vi "RT Loop - Analyze Acceleration_V2_CSV.vi"(7 "testing":bool, 8 "error in (no error)":errorcluster, 9 "Acceleration RT FIFO In":T2, 10 "FPGA VI Reference Out 2":refnum<k20>, 11 "Message Queue":refnum<queue>) -> (1 "Acceleration RT FIFO Out":T2)   [LabVIEW 2017]
doc: "Read and analyze acceleration waveform data from FPGA via DMA FIFO. If the acceleration is over the limit, then send the acceleration waveform data to the Log Data Loop."
uses:
  UI Error Handlers/support/Message Queue/Message Cluster.ctl
  controls/Acceleration RT FIFO Reference.ctl
  Control 1.ctl
  data_sav.ctl
  Globals/Global - All RT Loop Stop.vi
  <vilib>/Utility/file.llb/Write Delimited Spreadsheet (DBL).vi
  Globals/Global - Configuration Options.vi
  <vilib>/Utility/error.llb/Error Cluster From Error Code.vi
  <vilib>/rvi/errors/niLvFpgaAdjustHostInterfaceError.vi
  <vilib>/Utility/file.llb/Write Delimited Spreadsheet (string).vi
  <vilib>/rvi/interface/nirviMethod/nirviMethod.xnode
  <vilib>/FPGAPlugInAG/Dynamic/niLvFpga_ReadFifo_Dynamic.vi
  <vilib>/rvi/errors/niLvFpgaMergeErrorWithErrorCode.vi
  UI Error Handlers/support/Message Queue/Message Queue.lvlib
panel:
  out "size(s)":i32
  out "Cluster":cluster{"Array":T1[], "AVI Path":path}={"Array"=[], "AVI Path"=path "u:/data_log"}
  out "Free Physical Memory or Largest Contiguous Memory (bytes)":i64(graph)
  out "error out":errorcluster
  out "x-y":u32
  out "G1 status":cluster{"G1 trigger":bool}
  out "G1 status.G1 trigger":bool
  out "sta":bool
  out "logical OR":bool
  in  "Data Rate (Hz)":dbl
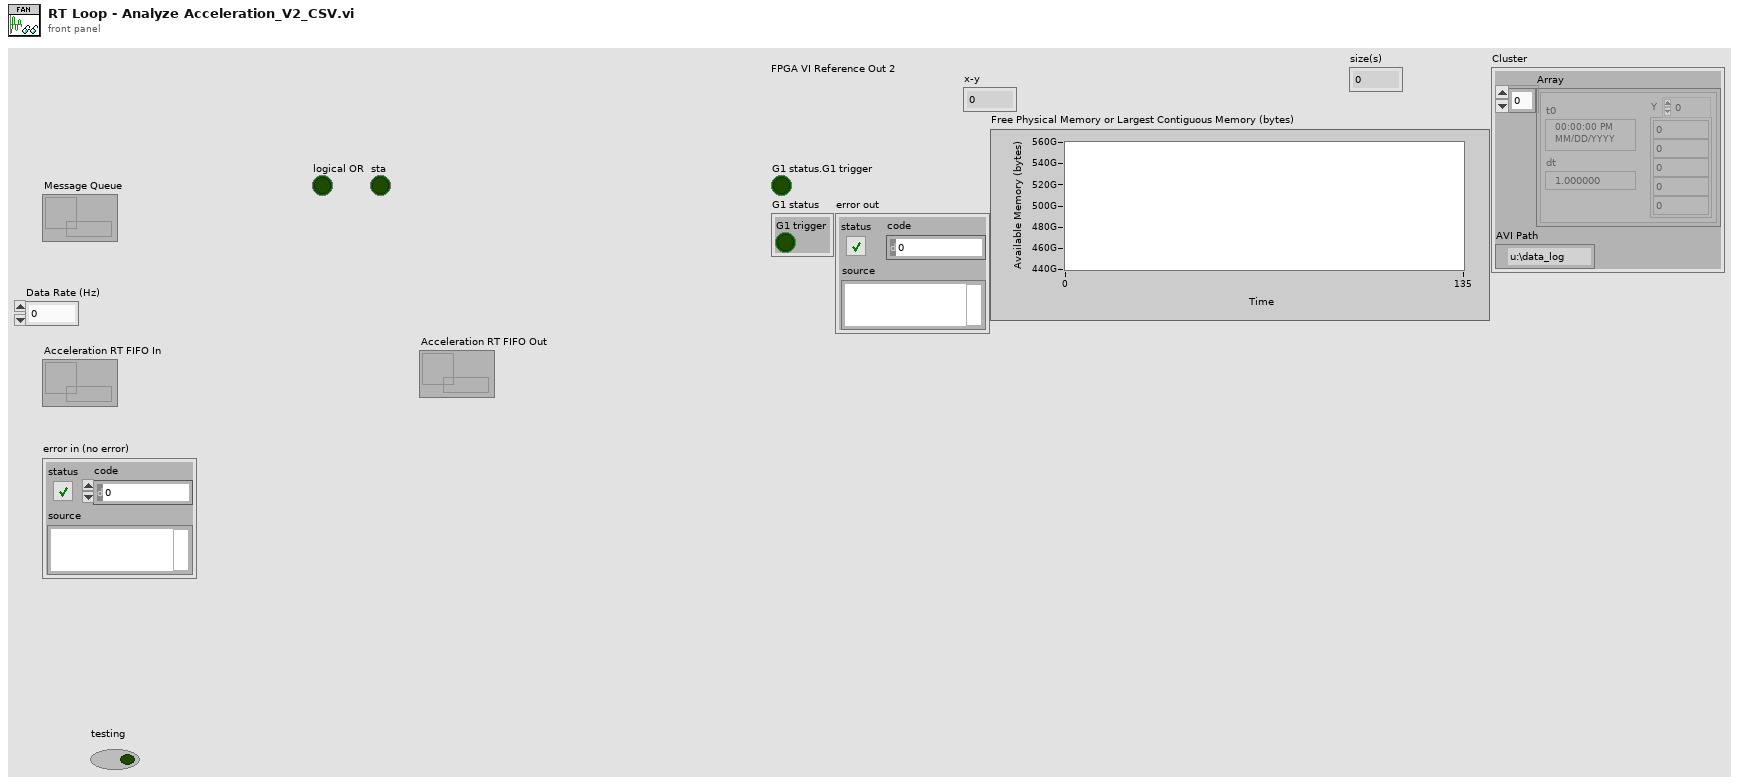
[diagram p1: front panel]
types:
  T1 = typedef "Control 1.ctl" = waveform(dbl)
  T2 = typedef "Acceleration RT FIFO Reference.ctl" = refnum<k33>
  T3 = typedef "data_sav.ctl" = cluster{"Log File out 2":refnum<k34>, "Array":T1[]}
  T4 = cluster{"Tool data":cluster{"Number of teeth":sgl}, "Cutting data":cluster{"rpm":sgl}, "Limits":cluster{"Magnitude threshold":sgl, "Tolerance":sgl}, "G1 status":cluster{"G1 trigger":bool}}
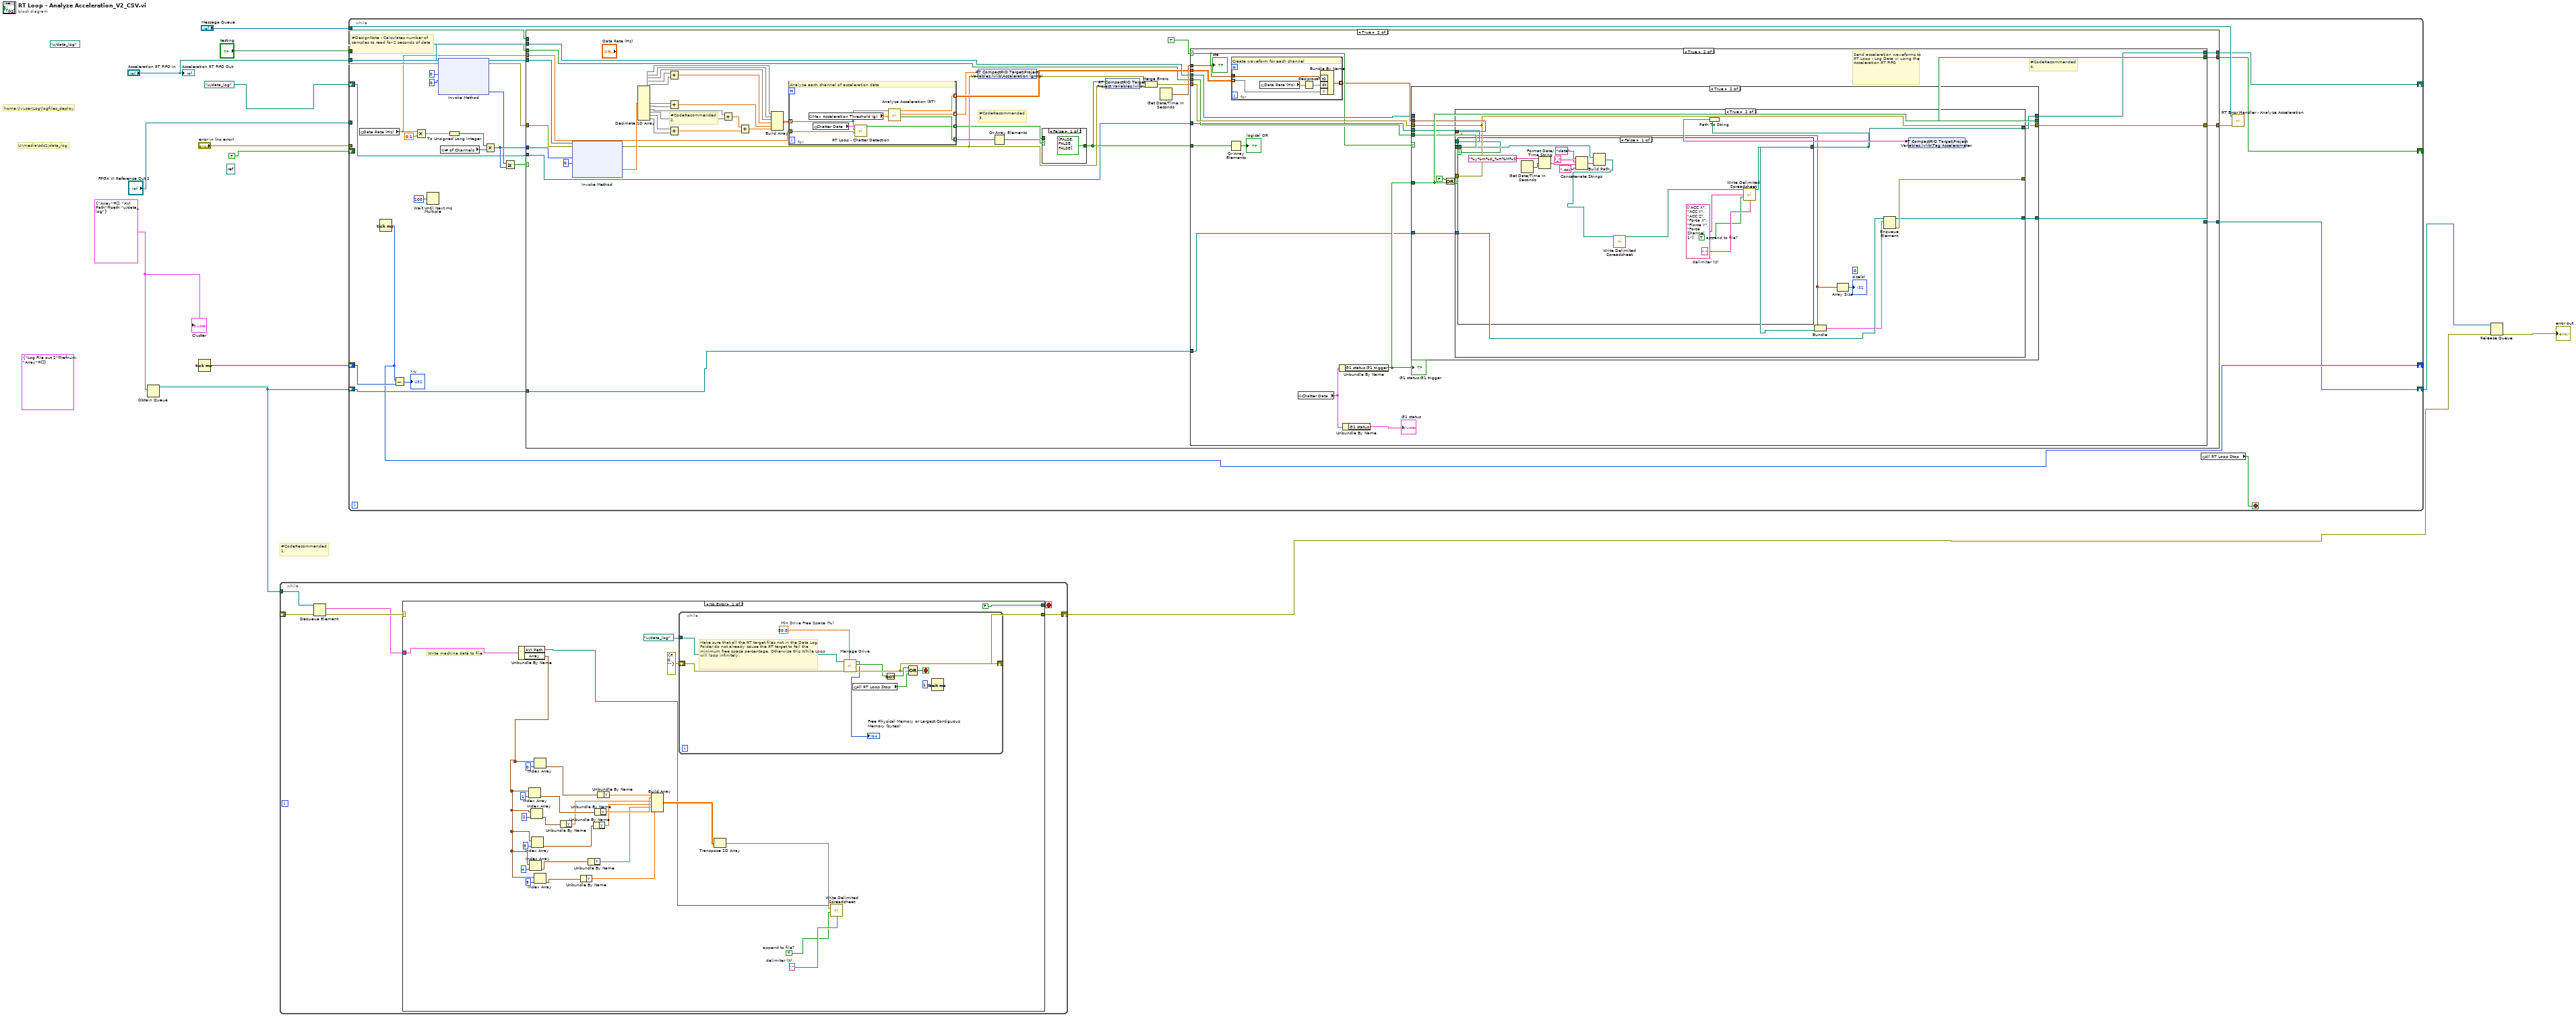
[diagram p0: block diagram]
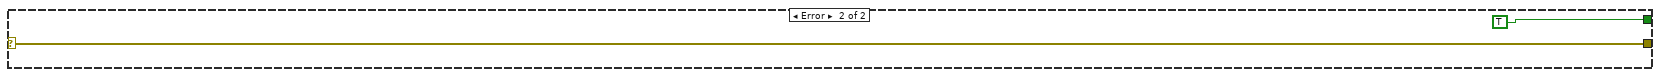
[diagram p2: hidden frame]
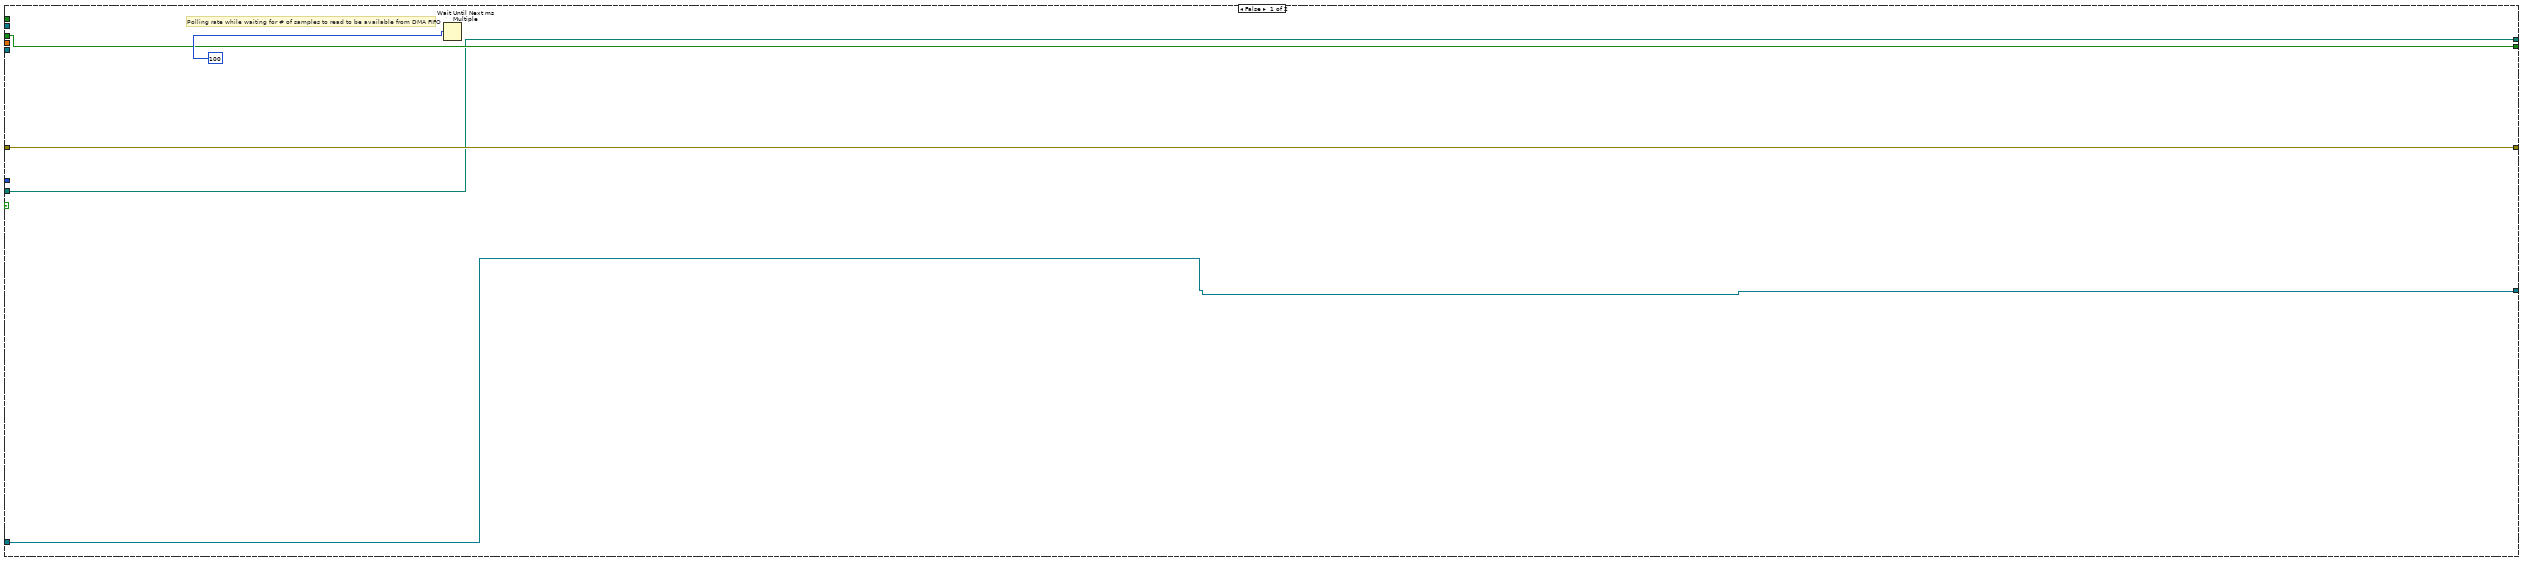
[diagram p3: hidden frame]
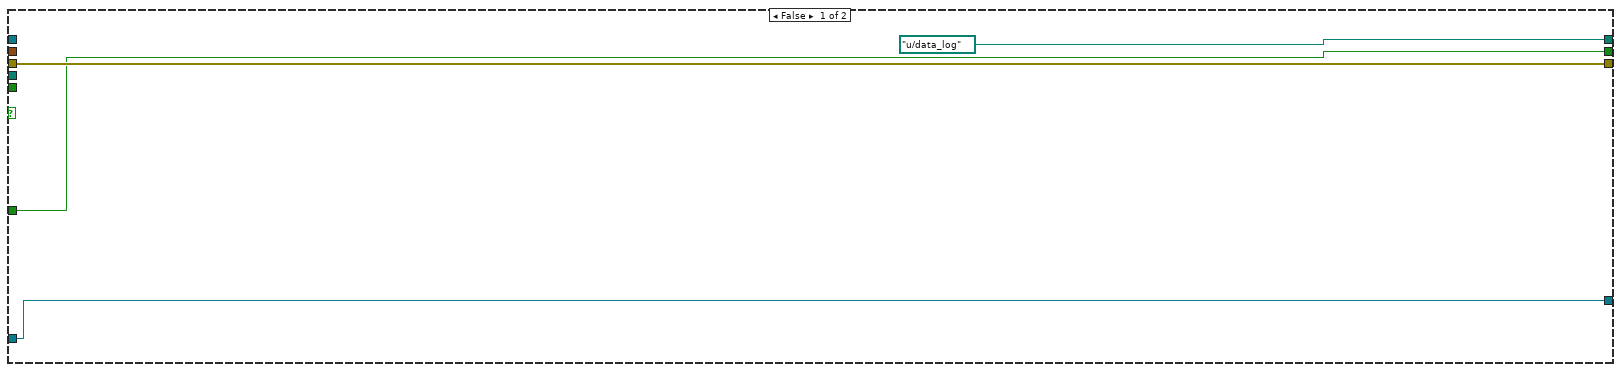
[diagram p6: hidden frame]
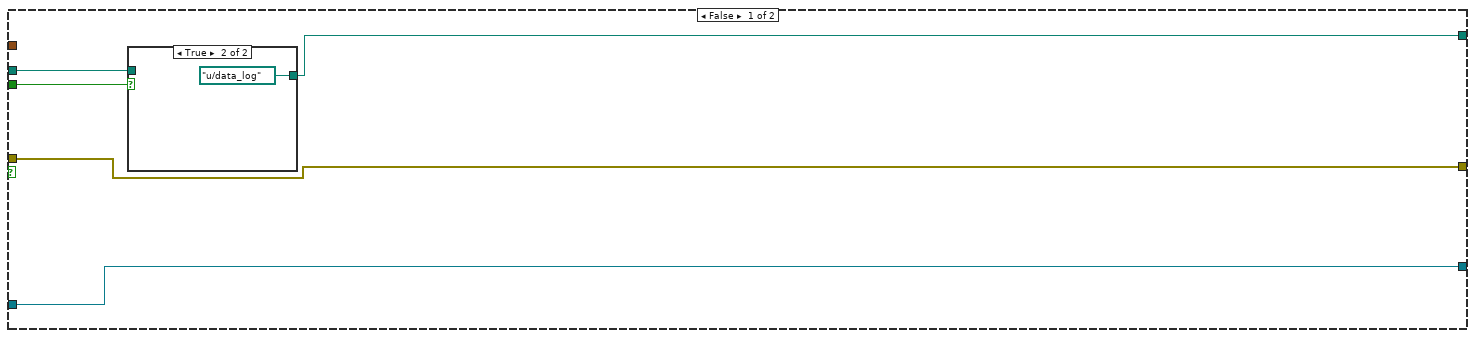
[diagram p7: hidden frame]
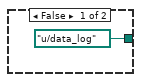
[diagram p8: hidden frame]
diagram:
  w1 = cluster{"Array":T1[], "AVI Path":path} {"Array"=[], "AVI Path"=path "u:/data_log"}
  (unwired) path "u:/data_log" ("AVI Path")
  (unwired) T3 {"Log File out 2"=refnum, "Array"=[]}
  (unwired) refnum<k34> refnum ("Log File out")
  # "U:\\media\\sdc1\\data_log"
  # "home:\\lvuser\\Log\\logfiles_deploy"
  # "#CodeRecommended\n1."
  n1 = Obtain Queue(element data type=w1) -> (queue out=w6:refnum<queue>)  [unwired: 4 in, 2 out]
  n2 = Tick Count (ms)() -> (millisecond timer value=w8:u32)
  n3 = while {
    tunnel: w6 -> [w19]
    shift-right: [w15] -> w4
    shift-left: _ -> [w18]
    stop <- w16 stop-if-true
    n4 = Dequeue Element(queue=w19, error in (no error)=w18) -> (element=w14:cluster{"Array":T1[], "AVI Path":path}, error out=w17:errorcluster)  [unwired: 1 in, 2 out]
    n5 = case shown="No Error" w17 {
      selector: w17 -> [_ w59]
      tunnel: [FALSE TRUE] -> w16
      tunnel: [w46 w59] -> w15
      tunnel: w14 -> [w45 _]
      frame No Error {
        w30 = TRUE  # append to file?
        w31 = ","  # delimiter (\t)
        # "Write machine data to file"
        n6 = Unbundle By Name(w45) -> ("AVI Path"=w20:path, "Array"=w32:T1[])
        n7 = Index Array(array=w32, index=1) -> (element=w37:T1)
        n8 = Index Array(array=w32, index=4) -> (element=w34:T1)
        n9 = Index Array(array=w32, index=2) -> (element=w28:T1)
        n10 = Index Array(array=w32, index=3) -> (element=w35:T1)
        n11 = Index Array(array=w32, index=0) -> (element=w42:T1)
        n12 = Index Array(array=w32, index=5) -> (element=w33:T1)
        n13 = Unbundle By Name(w28) -> ("Y"=w26:dbl[])
        n14 = Unbundle By Name(w33) -> ("Y"=w23:dbl[])
        n15 = Unbundle By Name(w34) -> ("Y"=w24:dbl[])
        n16 = Unbundle By Name(w35) -> ("Y"=w25:dbl[])
        n17 = Unbundle By Name(w37) -> ("Y"=w27:dbl[])
        n18 = Unbundle By Name(w42) -> ("Y"=w29:dbl[])
        n19 = Build Array(w29, w27, w26, w25, w24, w23) -> (w22:dbl[][])
        n20 = while {
          shift-right: [w53] -> w46
          shift-left: errorcluster {"status"=FALSE, "code"=0, "source"=""} ("error out") -> [w54]
          tunnel: path "u:/data_log" ("AVI Path") -> [w51]
          stop <- w58 stop-if-true
          w52 = 50.0  # Min Drive Free Space (%)
          # "Make sure that all the RT target files not in the Data Log Folder do not already cause the RT target to fail the minimum free space percentage. Otherwise this While Loop will loop infinitely."
          n21 = call "Manage Drive.vi"("Min Drive Free Space (%)"=w52, "error in"=w54, "Data Folder"=w51) -> ("error out"=w53:errorcluster, "Drive Space Below Limit"=w50:bool, "size (bytes)"=→"Free Physical Memory or Largest Contiguous Memory (bytes)":i64)  [unwired: 6 in]
          n22 = global read "Global - All RT Loop Stop.vi" "All RT Loop Stop"() -> (w55:bool)
          n23 = Not(x=w50) -> (.not. x?=w57:bool)
          n24 = Compound Arithmetic op=OR(w57, w53, w55) -> (w58:bool)
          n25 = Wait (ms)(milliseconds to wait=u32 1) -> ()  [unwired: 1 out]
        }
        n26 = Transpose 2D Array(2D array=w22) -> (transposed array=w21:dbl[][])
        n27 = call-poly <vilib>:"Write Delimited Spreadsheet.vi"("file path (dialog if empty)"=w20, "2D data"=w21, "append to file? (new file:F)"=w30, "delimiter (\\t)"=w31) -> ()  [unwired: 10 in, 2 out]
      }
      frame Error {
      }
    }
  }
  n28 = while {
    tunnel: "FPGA VI Reference Out 2" -> [w89]
    tunnel: "error in (no error)" -> [w88]
    tunnel: "Message Queue" -> [w81]
    tunnel: "Acceleration RT FIFO In" -> [w79]
    tunnel: "testing" -> [w71]
    shift-right: [w68] -> _
    shift-left: path "u:/data_log" ("AVI Path") -> [w67]
    shift-right: [w70] -> _
    shift-left: FALSE -> [w69]
    shift-right: [w65] -> _
    shift-left: w8 -> [w66]
    shift-right: [w62] -> w5
    shift-left: w6 -> [w63]
    stop <- w82 stop-if-true
    # "#DesignNote - Calculates number of samples to read for 2 seconds of data"
    n29 = global read "Global - Configuration Options.vi" "Data Rate (Hz)"() -> (w73:dbl)
    n30 = Tick Count (ms)() -> (millisecond timer value=w65:u32)
    n31 = Subtract(x=w65, y=w66) -> (x-y=→"x-y":u32)
    n32 = Multiply(x=w73, y=0.1) -> (x*y=w77:dbl)
    n33 = Wait Until Next ms Multiple(millisecond multiple=u32 100) -> ()  [unwired: 1 out]
    n34 = xnode "Invoke Method"("FPGA VI Reference In"=w89, "error in"=w88, "Number of Elements"=u32 0, "Timeout (ms)"=0) -> ("FPGA VI Reference Out"=w85:refnum<k20>, "error out"=w84:errorcluster, "Elements Remaining"=w72:u32)  [unwired: 1 out]
    n35 = global read "Global - Configuration Options.vi" "# of Channels"() -> (w74:u32)
    n36 = To Unsigned Long Integer(number=w77) -> (unsigned 32bit integer=w76:u32)
    n37 = Multiply(x=w76, y=w74) -> (x*y=w75:u32)
    n38 = Greater Or Equal?(x=w72, y=w75) -> (x >= y?=w83:bool)
    n39 = case shown="True" w83 {
      tunnel: w85 -> [_ w137]
      tunnel: w84 -> [w94 w136]
      tunnel: [w94 w132] -> w80
      tunnel: w75 -> [_ w135]
      tunnel: w79 -> [_ w130]
      tunnel: w73 -> [_ w126]
      tunnel: w71 -> [_ _]
      tunnel: [w92 w118] -> w70
      tunnel: w69 -> [w92 w117]
      tunnel: [w91 w116] -> w68
      tunnel: w67 -> [w91 w115]
      tunnel: w63 -> [w90 w96]
      tunnel: [w90 w95] -> w62
      frame False {
        # "Polling rate while waiting for # of samples to read to be available from DMA FIFO"
        n40 = Wait Until Next ms Multiple(millisecond multiple=u32 100) -> ()  [unwired: 1 out]
      }
      frame True {
        # "#CodeRecommended\n3."
        # "#CodeRecommended\n2."
        n41 = xnode "Invoke Method"("FPGA VI Reference In"=w137, "error in"=w136, "Number of Elements"=w135, "Timeout (ms)"=0) -> ("error out"=w125:errorcluster, "Data"=w129:sgl[])  [unwired: 2 out]
        n42 = Decimate 1D Array(w129) -> (w112:sgl[], w111:sgl[], w110:sgl[], w109:sgl[], w108:sgl[], w106:sgl[], w105:sgl[], w104:sgl[], w103:sgl[], w102:sgl[], w101:sgl[])
        n43 = Add(x=w109, y=w108) -> (x+y=w107:sgl[])
        n44 = Add(x=w106, y=w105) -> (x+y=w97:sgl[])
        n45 = Add(x=w102, y=w101) -> (x+y=w99:sgl[])
        n46 = Add(x=w104, y=w103) -> (x+y=w100:sgl[])
        n47 = Add(x=w100, y=w99) -> (x+y=w98:sgl[])
        n48 = Build Array(w112, w111, w110, w107, w97, w98) -> (w113:sgl[][])
        n49 = for {
          tunnel: [w147] -> w131 mode=indexing
          tunnel: [w146] -> w128 mode=indexing
          tunnel: [w145] -> w127 mode=indexing
          tunnel: w126 -> [w143]
          tunnel: [w142] -> w120 mode=indexing
          tunnel: w113 -> [w140] mode=indexing
          # "Analyze each channel of acceleration data"
          n50 = global read "Global - Configuration Options.vi" "Max Acceleration Threshold (g)"() -> (w144:sgl)
          n51 = global read "Global - Configuration Options.vi" "Chatter Data"() -> (w141:T4)
          n52 = call "RT Loop - Chatter Detection.vi"("Data Rate (Hz)"=w143, "Acceleration Waveform (SGL)"=w140, "Chatter Data"=w141) -> ("Chatter?"=w142:bool)  [unwired: 8 in]
          n53 = call "Analyze Acceleration (RT).vi"("Max Instantaneous Acceleration (g)"=w144, "Acceleration Waveform (SGL)"=w140) -> ("Over Limit?"=w147:bool, "Acceleration (grms)"=w145:dbl, "Acceleration Waveform (DBL)"=w146:dbl[])  [unwired: 7 in]
        }
        n54 = shared-variable "RT CompactRIO Target\\Project Variables.lvlib\\Acceleration (grms)"(w127, error in=w125) -> (error out=w123:errorcluster)
        n55 = Or Array Elements(Boolean array=w131) -> (logical OR=w121:bool)
        n56 = case shown="False" w121 {
          tunnel: w120 -> [_ w139]
          tunnel: [bool[] [FALSE, FALSE, FALSE] ("Chatter?") w139] -> w119
          frame False {
          }
          frame True {
          }
        }
        n57 = shared-variable "RT CompactRIO Target\\Project Variables.lvlib\\Chatter?"(w119, error in=w125) -> (error out=w124:errorcluster)
        n58 = Merge Errors(w123, w124) -> (w122:errorcluster)
        n59 = Get Date/Time In Seconds() -> (seconds since 1Jan1904=w133:timestamp)
        n60 = case shown="True" TRUE {
          selector: TRUE -> [_ w152]
          tunnel: w133 -> [_ w169]
          tunnel: w122 -> [w151 w168]
          tunnel: [w151 w155] -> w132
          tunnel: w130 -> [_ w166]
          tunnel: w128 -> [_ w165]
          tunnel: w119 -> [_ w163]
          tunnel: [w150 w160] -> w118
          tunnel: w117 -> [w150 w159]
          tunnel: [w149 w158] -> w116
          tunnel: w115 -> [w149 w156]
          tunnel: w96 -> [w148 w154]
          tunnel: [w148 w153] -> w95
          frame False {
          }
          frame True {
            # "#CodeRecommended\n4."
            # "Send acceleration waveforms to RT Loop - Log Data.vi using the Acceleration RT FIFO"
            n61 = Or Array Elements(Boolean array=w163) -> (logical OR=→"logical OR":bool)
            n62 = for {
              tunnel: w165 -> [w220] mode=indexing
              tunnel: w169 -> [w219]
              tunnel: [w217] -> w167 mode=indexing
              # "Create waveform for each channel"
              n63 = global read "Global - Configuration Options.vi" "Data Rate (Hz)"() -> (w216:dbl)
              n64 = Reciprocal(x=w216) -> (1/x=w218:dbl)
              n65 = Bundle By Name("t0"=w219, "dt"=w218, "Y"=w220) -> (w217:waveform(dbl))  [unwired: 1 in]
            }
            n66 = global read "Global - Configuration Options.vi" "Chatter Data"() -> (w162:T4)
            n67 = Unbundle By Name(w162) -> ("G1 status.G1 trigger"=w157:bool)
            "G1 status.G1 trigger" <- w157
            n68 = Unbundle By Name(w162) -> ("G1 status"=→"G1 status":cluster{"G1 trigger":bool})
            n69 = case shown="True" w152 {
              tunnel: w168 -> [w173 w176]
              tunnel: w167 -> [_ w177]
              tunnel: w166 -> [_ _]
              tunnel: w157 -> [w172 w181]
              tunnel: [w172 w181] -> w160
              tunnel: w159 -> [_ w180]
              tunnel: [path "u:/data_log" ("AVI Path") w179] -> w158
              tunnel: w156 -> [_ w178]
              tunnel: [w173 w176] -> w155
              tunnel: w154 -> [w170 w174]
              tunnel: [w170 w175] -> w153
              frame False {
              }
              frame True {
                n70 = Or(x=FALSE, y=w181) -> (x .or. y?=w183:bool)
                n71 = case shown="True" w183 {
                  tunnel: w178 -> [w186 w200]
                  tunnel: [w188 w194] -> w179
                  tunnel: w180 -> [w187 w199]
                  tunnel: w177 -> [_ w192]
                  tunnel: w176 -> [w185 _]
                  tunnel: [w185 w197] -> _
                  tunnel: w174 -> [w184 w195]
                  tunnel: [w184 w196] -> w175
                  frame False {
                    n72 = case shown="True" w187 {
                      tunnel: [path "u:/data_log" ("AVI Path") path "u:/data_log" ("AVI Path")] -> w188
                      tunnel: w186 -> [_ _]
                      frame False {
                      }
                      frame True {
                      }
                    }
                  }
                  frame True {
                    (unwired) 0 ("size(s)")
                    n73 = case shown="False" w199 {
                      tunnel: w200 -> [w207 w215]
                      tunnel: [w201 w215] -> w194
                      frame False {
                        w204 = TRUE  # append to file?
                        w205 = ","  # delimiter (\t)
                        n74 = Get Date/Time In Seconds() -> (seconds since 1Jan1904=w210:timestamp)
                        n75 = Format Date/Time String(time format string (%c)="%y%m%d_%H%M%S", seconds (now)=w210) -> (date/time string=w213:string)  [unwired: 1 out]
                        n76 = Concatenate Strings("data" ("string"), "_" ("string"), w213, ".csv" ("string")) -> (w208:string)
                        n77 = Build Path(base path=w207, name or relative path=w208) -> (appended path=w202:path)
                        n78 = call-poly <vilib>:"Write Delimited Spreadsheet.vi"("file path (dialog if empty)"=w202) -> ("new file path (Not A Path if cancelled)"=w203:path)  [unwired: 13 in, 1 out]
                        n79 = call-poly <vilib>:"Write Delimited Spreadsheet.vi"("file path (dialog if empty)"=w203, "1D data"=string[] ["ACC X", "ACC Y", "ACC Z", "Force X", "Fiorce Y", "Force Zhannel 1"] ("Channel Names"), "append to file? (new file:F)"=w204, "delimiter (\\t)"=w205) -> ("new file path (Not A Path if cancelled)"=w201:path)  [unwired: 10 in, 1 out]
                      }
                      frame True {
                      }
                    }
                    n80 = Path To String(path=w194) -> (string=w198:string)
                    n81 = Bundle(w192, "AVI Path"=w194) -> (w193:cluster{waveform(dbl)[], "AVI Path":path})  [unwired: 1 in]
                    n82 = Array Size(array=w192) -> (size(s)=→"size(s)":i32)
                    n83 = Enqueue Element(queue=w195, element=w193) -> (queue out=w196:refnum<queue>, error out=w197:errorcluster)  [unwired: 2 in, 1 out]
                    n84 = shared-variable "RT CompactRIO Target\\Project Variables.lvlib\\Tag Accelerometer"(w198) -> ()  [unwired: 1 in, 1 out]
                  }
                }
              }
            }
            "sta" <- w152
          }
        }
      }
    }
    n85 = global read "Global - All RT Loop Stop.vi" "All RT Loop Stop"() -> (w82:bool)
    n86 = call "RT Error Handler - Analyze Acceleration.vi"("error in (no error)"=w80, "Message Queue"=w81) -> ()  [unwired: 9 in, 1 out]
  }
  n87 = Release Queue(queue=w5, error in (no error)=w4) -> (error out=→"error out":errorcluster)  [unwired: 1 in, 2 out]
  "Acceleration RT FIFO Out" <- "Acceleration RT FIFO In"
  "Cluster" <- w1
